vi "SendExit.vi"(8 "error in (no error)":errorcluster, 11 "DownStreamMsgHandler in":refnum<class "DownStreamMsgHandler.lvclass">) -> (0 "error out":errorcluster, 3 "DownStreamMsgHandler out":refnum<class "DownStreamMsgHandler.lvclass">)   [LabVIEW 2020, in "DownstreamMsgHandler.lvlib" / "DownStreamMsgHandler.lvclass"]
uses:
  DownStreamMsgHandler.lvclass
  UpstreamMsg/Exit/Exit.lvclass
  C:/Users/taylo/Projects/g-go-service-fwrk/scratchpad/ServiceManagerBeta/ServiceManager/UpstreamMsg/UpstreamMsgParent/UpstreamMsgParent.lvclass
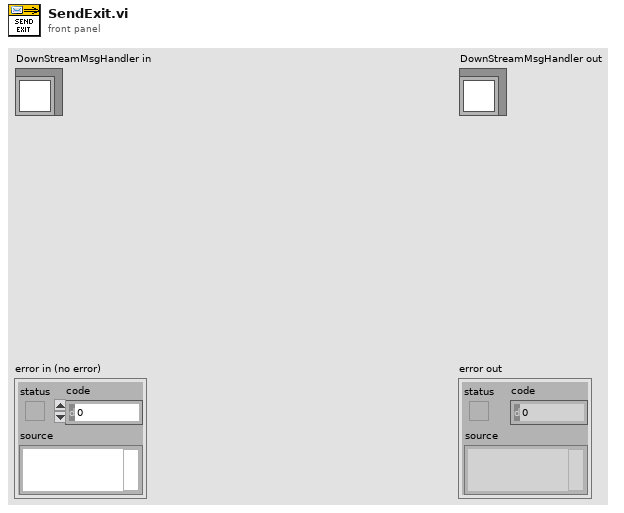
[diagram p1: front panel]
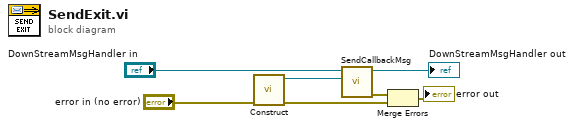
[diagram p0: block diagram]
diagram:
  n1 = call "Construct.vi"("error in (no error)"="error in (no error)") -> ("error out"=w1:errorcluster, "Exit out"=w4:refnum<class "Exit.lvclass">)  [unwired: 9 in]
  n2 = call-dynamic "SendCallbackMsg.vi"("UpstreamMsg"=w4, "DownStreamMsgHandler in"="DownStreamMsgHandler in") -> ("error out"=w5:errorcluster, "DownStreamMsgHandler out"=→"DownStreamMsgHandler out":refnum<class "DownStreamMsgHandler.lvclass">)  [unwired: 8 in]
  n3 = Merge Errors(w5, w1) -> (→"error out":errorcluster)
